vi "timing (SubVI).vi"(8 "Enum F":T1, 9 "Enum T":T1, 10 "red sec":i32, 11 "Numeric in":i32) -> (2 "Enum out":T1, 3 "Numeric out":i32)   [LabVIEW 2019]
uses:
  control/Control 1.ctl
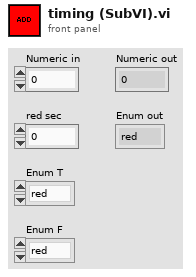
[diagram p1: front panel]
types:
  T1 = typedef "Control 1.ctl" = enum16{"red", "yellow", "green"}
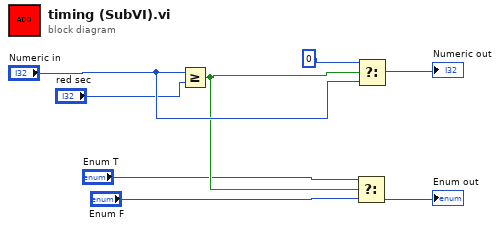
[diagram p0: block diagram]
diagram:
  n1 = Greater Or Equal?(x="Numeric in", y="red sec") -> (x >= y?=w7:bool)
  n2 = Select(t="Enum T", s=w7, f="Enum F") -> (s? t:f=→"Enum out":T1)
  n3 = Select(t=0, s=w7, f="Numeric in") -> (s? t:f=→"Numeric out":i32)
